vi "Decimate array by factor.vi"(9 "Input array in":sgl[](array[numeric]), 10 "Decimation factor":i32, 11 "Decimaion method":T1(ring)) -> (3 "Array":sgl[](array[numeric]))   [LabVIEW 2021, in "MatS Libs.lvlib"]
uses:
  <userlib>/MatS Libs/MatS Libs.lvlib
  <vilib>/GPower/Math/Library/Stat/Median/MedianSGL.vi
  <userlib>/_MGI/1D Array/MGI Average/MGI Average (SGL[]).vi
  <vilib>/GPower/Math/GPMath.lvlib
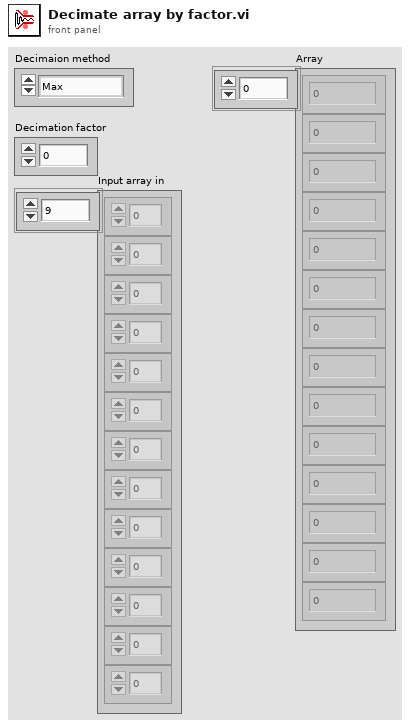
[diagram p1: front panel]
types:
  T1 = enum16{"Max", "Min", "Median", "Average", "First", "Last"}
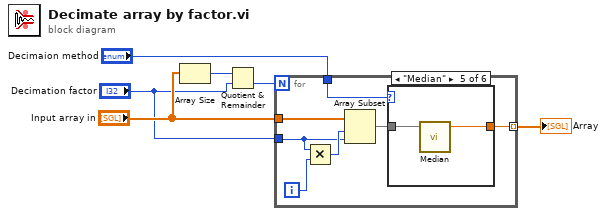
[diagram p0: block diagram]
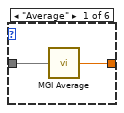
[diagram p2: hidden frame]
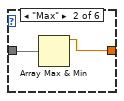
[diagram p3: hidden frame]
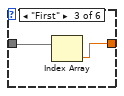
[diagram p4: hidden frame]
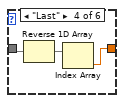
[diagram p5: hidden frame]
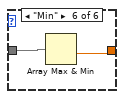
[diagram p6: hidden frame]
diagram:
  n1 = Array Size(array="Input array in") -> (size(s)=w1:i32)
  n2 = Quotient & Remainder(x=w1, y="Decimation factor") -> (floor(x/y)=w2:i32)  [unwired: 1 out]
  n3 = for {
    N: w2 -> [_]
    tunnel: "Decimation factor" -> [w11]
    tunnel: "Input array in" -> [w13]
    tunnel: [w8] -> w5 mode=indexing
    tunnel: "Decimaion method" -> [w7]
    i -> [w10]
    n4 = Multiply(x=w11, y=w10) -> (x*y=w12:i32)
    n5 = Array Subset(array=w13, index=w12, length=w11) -> (w9:sgl[])
    n6 = case shown="\"Median\"" w7 {
      tunnel: w9 -> [w15 w17 w19 w22 w24 w26]
      tunnel: [w14 w16 w18 w21 w23 w25] -> w8
      frame "Average" {
        n7 = call-poly <userlib>:"MGI Average.vi"("Single[]"=w15) -> ("Average"=w14:sgl)  [unwired: 1 in]
      }
      frame "Max" {
        n8 = Array Max & Min(array=w17) -> (max value=w16:sgl)  [unwired: 3 out]
      }
      frame "First" {
        n9 = Index Array(array=w19) -> (element=w18:sgl)  [unwired: 1 in]
      }
      frame "Last" {
        n10 = Reverse 1D Array(array=w22) -> (reversed array=w20:sgl[])
        n11 = Index Array(array=w20) -> (element=w21:sgl)  [unwired: 1 in]
      }
      frame "Median" {
        n12 = call-poly <vilib>:"Median.vi"("X"=w24) -> ("Median"=w23:sgl)  [unwired: 4 in]
      }
      frame "Min" {
        n13 = Array Max & Min(array=w26) -> (min value=w25:sgl)  [unwired: 3 out]
      }
    }
  }
  "Array" <- w5
